vi "Start.vi"(4 "Manual thread":i64, 6 "Thread":T1[](array[typedef]), 7 "domainName":string, 8 "error in (no error)":errorcluster, 9 "password":string, 10 "userName":string, 11 "Impersonate in":refnum<class "LogonUser.lvclass">) -> (0 "error out":errorcluster, 3 "Impersonate out":refnum<class "LogonUser.lvclass">)   [LabVIEW 2018, in "LogonUser.lvclass"]
doc: "©2019\nWiebe Walstra\nwww.carya.nl"
uses:
  LogonUser.lvclass
  Threads.ctl
  <vilib>/Platform/TimedLoop/XDataNode/timing_clust.ctl
  <vilib>/Platform/TimedLoop/XDataNode/nitl_modes.ctl
  <vilib>/Platform/TimedLoop/XDataNode/wakeup.ctl
  LogonUser.lvclass/LogonUser.ctl
  <vilib>/Utility/error.llb/Error Cluster From Error Code.vi
  <vilib>/Platform/TimedLoop/XDataNode/XDataNode.xnode
  advapi32.dll
  kernel32.dll
  <vilib>/Platform/TimedLoop/XDataNode/XDNodeRunTimeDep.lvlib
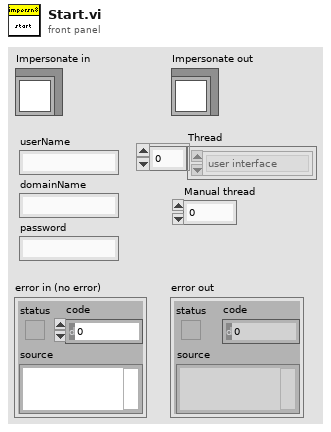
[diagram p1: front panel]
types:
  T1 = typedef "LogonUser.lvclass/Threads.ctl" = enum32{"user interface", "standard", "instrument i/o", "data acquisition", "other 1", "other 2", "same as caller", "manual"}
  T2 = typedef "XDNodeRunTimeDep.lvlib/timing_clust.ctl" = cluster{"Expected End [f-1]":u64, "Actual End [f-1]":u64, "Finished Late? [f-1]":bool, "Expected End [i-1]":u64, "Actual End [i-1]":u64, "Finished Late? [i-1]":bool, "Expected Start [i]":u64, "Actual Start [i]":u64, "Expected Start [f]":u64, "Actual Start [f]":u64, "Source Name":string, "Structure Name":string, "Period":i64, "Deadline":i64, "Offset":i64, "Start":i64, "Priority":i32, "Timeout":i32, "Mode":T3, "Wakeup Reason":T4, "Error":errorcluster, "Source Type":string, "Secondary Source Type":string, "Global End Time":u64, "Global Start Time":u64, "Frame Duration":u64, "Iteration Duration":u64, "Assigned CPU":i32, "I/O Scan Engine Mode":u32}
  T3 = typedef "XDNodeRunTimeDep.lvlib/nitl_modes.ctl" = enum32{"No Change", "Process missed periods, maintain original phase", "Discard missed periods, maintain original phase", "Process missed periods, ignore original phase", "Discard missed periods, ignore original phase"}
  T4 = typedef "XDNodeRunTimeDep.lvlib/wakeup.ctl" = enum32{"Normal", "Aborted", "Asynchronous wakeup", "Timing source error", "Timed loop error", "Timeout"}
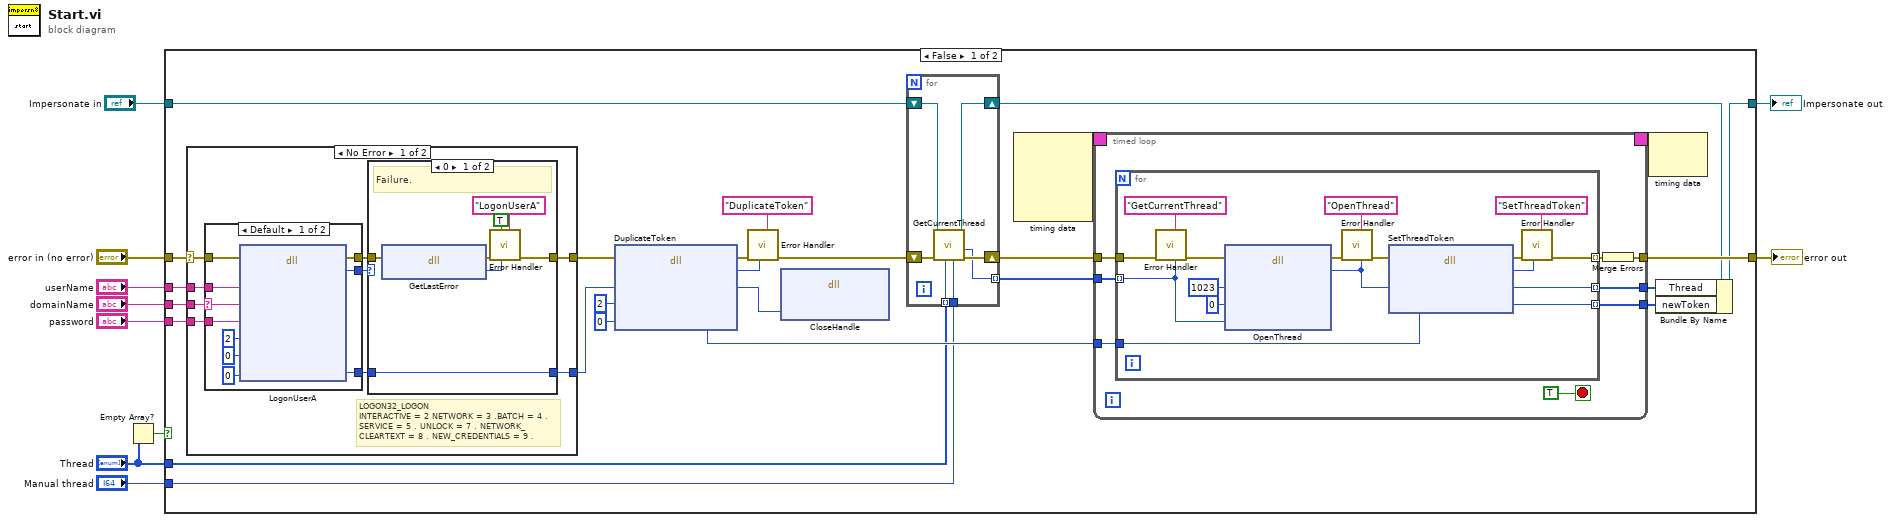
[diagram p0: block diagram]
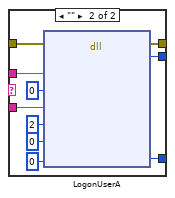
[diagram p2: hidden frame]
diagram:
  n1 = Empty Array?(array="Thread") -> (empty?=w3:bool)
  n2 = case shown="False" w3 {
    tunnel: [w14 w113] -> w10
    tunnel: "userName" -> [w33 _]
    tunnel: "password" -> [w32 _]
    tunnel: "error in (no error)" -> [w31 w112]
    tunnel: [w28 w112] -> w6
    tunnel: "Impersonate in" -> [w20 w113]
    tunnel: "Thread" -> [w19 _]
    tunnel: "Manual thread" -> [w11 _]
    tunnel: "domainName" -> [w12 _]
    frame False {
      n3 = case shown="No Error" w31 {
        selector: w31 -> [w69 w103]
        tunnel: w33 -> [w71 _]
        tunnel: w32 -> [w70 _]
        tunnel: [w67 w103] -> w30
        tunnel: [w66 _] -> w27
        tunnel: w12 -> [w65 _]
        frame No Error {
          # "LOGON32_LOGON \nINTERACTIVE = 2 NETWORK = 3 .BATCH = 4 . SERVICE = 5 . UNLOCK = 7 . NETWORK_CLEARTEXT = 8 . NEW_CREDENTIALS = 9 ."
          n4 = case shown="Default" w65 {
            selector: w65 -> [w75 _]
            tunnel: [w83 w93] -> w73
            tunnel: [w80 w90] -> w72
            tunnel: w71 -> [w79 w88]
            tunnel: w70 -> [w74 w87]
            tunnel: w69 -> [w78 w86]
            tunnel: [w77 w85] -> w68
            frame Default {
              n5 = dll-call lib="advapi32.dll" fn="LogonUserA"(error in=w78, "username"=w79, "domain"=w75, "password"=w74, "dwLogonType"=2, "dwLogonProvider"=0 ("dwLogonType"), "phToken"=i64 0) -> (error out=w77:errorcluster, "success"=w80:i32, "phToken"=w83:i64)  [unwired: 7 in, 1 out]
            }
            frame "" {
              n6 = dll-call lib="advapi32.dll" fn="LogonUserA"(error in=w86, "username"=w88, "domain"=0, "password"=w87, "dwLogonType"=2, "dwLogonProvider"=0 ("dwLogonType"), "phToken"=i64 0) -> (error out=w85:errorcluster, "success"=w90:i32, "phToken"=w93:i64)  [unwired: 7 in, 1 out]
            }
          }
          n7 = case shown="0" w72 {
            tunnel: w73 -> [w100 w102]
            tunnel: [w100 w102] -> w66
            tunnel: w68 -> [w99 w101]
            tunnel: [w97 w101] -> w67
            frame 0 {
              # "Failure."
              n8 = dll-call lib="kernel32.dll" fn="GetLastError"(error in=w99) -> (error out=w98:errorcluster, "error"=w96:i32)  [unwired: 2 in, 1 out]
              n9 = call "Error Handler.vi"("Label"="LogonUserA", "Error I32 [0]"=w96, "Error if 0? [T]"=TRUE ("Error if !0 [F, error if 0]"), "error in (no error)"=w98) -> ("error out"=w97:errorcluster)  [unwired: 7 in]
            }
            frame Default {
              # "Success."
            }
          }
        }
        frame Error {
        }
      }
      n10 = dll-call lib="advapi32.dll" fn="DuplicateToken"(error in=w30, "phToken"=w27, "impersonationLevel"=2, "newToken"=i64 0) -> (error out=w29:errorcluster, "success"=w26:i32, "phToken"=w34:i64, "newToken"=w24:i64)  [unwired: 3 in, 1 out]
      n11 = call "Error Handler.vi"("Label"="DuplicateToken", "Error I32 [0]"=w26, "error in (no error)"=w29) -> ("error out"=w13:errorcluster)  [unwired: 8 in]
      n12 = dll-call lib="kernel32.dll" fn="CloseHandle"("handle"=w34) -> ()  [unwired: 5 in, 2 out]
      n13 = for {
        shift-right: [w109] -> w21
        shift-left: w13 -> [w110]
        shift-right: [w107] -> w15
        shift-left: w20 -> [w108]
        tunnel: w19 -> [w106] mode=indexing
        tunnel: [w105] -> w18 mode=indexing
        tunnel: w11 -> [w104]
        n14 = call-dynamic "GetCurrentThread.vi"("Manual thread"=w104, "Thread"=w106, "error in (no error)"=w110, "Impersonate in"=w108) -> ("error out"=w109:errorcluster, "thread id"=w105:i64, "Impersonate out"=w107:refnum<class "LogonUser.lvclass">)  [unwired: 5 in]
      }
      n15 = node-c288() -> (w23:T2)  [unwired: 4 in]
      n16 = timed-loop {
        timing: w23 -> [_]
        timing-out: [_] -> w22
        tunnel: w24 -> [w42]
        tunnel: w18 -> [w40]
        tunnel: [w39] -> w17
        tunnel: [w38] -> w16
        tunnel: w21 -> [w43]
        tunnel: [w37] -> w28
        stop <- TRUE stop-if-true
        n17 = for {
          tunnel: w42 -> [w61]
          tunnel: [w60] -> w38 mode=indexing
          tunnel: [w59] -> w39 mode=indexing
          tunnel: w40 -> [w46] mode=indexing
          tunnel: w43 -> [w45]
          tunnel: [w49] -> w44 mode=indexing
          n18 = call "Error Handler.vi"("Error I64 [0]"=w46, "Label"="GetCurrentThread", "error in (no error)"=w45) -> ("error out"=w56:errorcluster)  [unwired: 8 in]
          n19 = dll-call lib="kernel32.dll" fn="OpenThread"(error in=w56, "dwDesiredAccess"=1023 ("bInheritHandle"), "bInheritHandle"=0, "ThreadID"=w46) -> (error out=w53:errorcluster, "thread"=w51:i64)  [unwired: 5 in, 1 out]
          n20 = call "Error Handler.vi"("Error I64 [0]"=w51, "Label"="OpenThread", "error in (no error)"=w53) -> ("error out"=w52:errorcluster)  [unwired: 8 in]
          n21 = dll-call lib="Advapi32.dll" fn="SetThreadToken"(error in=w52, "pThread"=w51, "newToken"=w61) -> (error out=w50:errorcluster, "success"=w48:i32, "pThread"=w59:i64, "newToken"=w60:i64)  [unwired: 2 in, 1 out]
          n22 = call "Error Handler.vi"("Label"="SetThreadToken", "Error I32 [0]"=w48, "error in (no error)"=w50) -> ("error out"=w49:errorcluster)  [unwired: 8 in]
        }
        n23 = Merge Errors(w44) -> (w37:errorcluster)
      }
      n24 = node-c288(w22) -> ()  [unwired: 1 out]
      n25 = Bundle By Name(cluster=w15, "Thread"=w17, "newToken"=w16) -> (w14:refnum<class "LogonUser.lvclass">)
    }
    frame True {
    }
  }
  "error out" <- w6
  "Impersonate out" <- w10
